vi "AddUniqueSubscription.vi"(0 "activeSubscriptions":T1[](array[typedef]), 2 "subscription":T1) -> (14 "activeSubscriptions":T1[](array[typedef]))   [LabVIEW 2017, in "STOMP.lvclass"]
uses:
  STOMP.lvclass
  Typedefs/Type_ActiveSubscription.ctl
  Typedefs/Type_AckHeader.ctl
  Typedefs/Type_FrameHeader.ctl
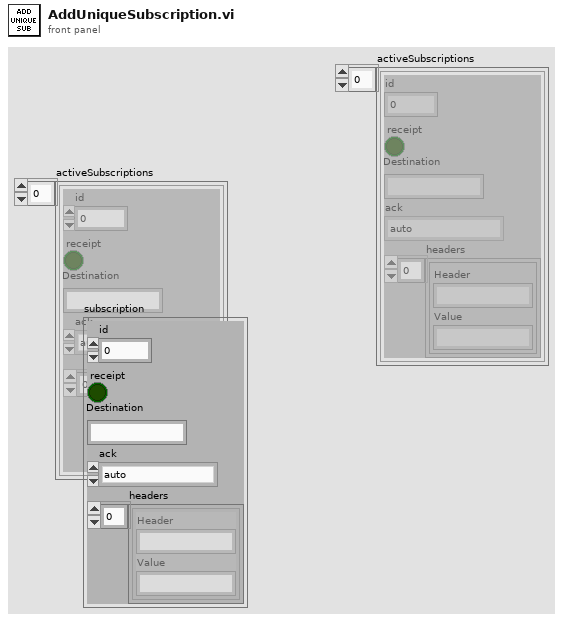
[diagram p1: front panel]
types:
  T1 = typedef "STOMP.lvclass/Type_ActiveSubscription.ctl" = cluster{"id":u64, "receipt":bool, "Destination":string, "ack":T2, "headers":T3[]}
  T2 = typedef "STOMP.lvclass/Type_AckHeader.ctl" = enum16{"auto", "client", "client-individual"}
  T3 = typedef "STOMP.lvclass/Type_FrameHeader.ctl" = cluster{"Header":string, "Value":string}
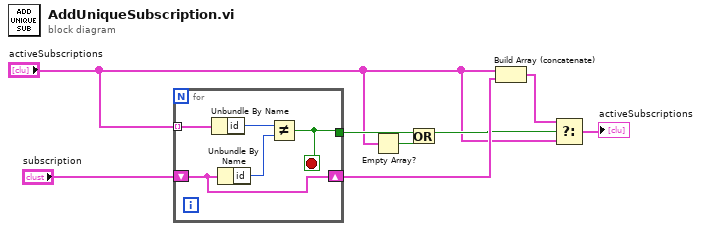
[diagram p0: block diagram]
diagram:
  n1 = for {
    tunnel: "activeSubscriptions" -> [w13] mode=indexing
    tunnel: [w10] -> w7
    shift-right: [w9] -> w6
    shift-left: "subscription" -> [w9]
    stop <- w10 stop-if-true
    n2 = Unbundle By Name(w13) -> ("id"=w12:u64)
    n3 = Unbundle By Name(w9) -> ("id"=w11:u64)
    n4 = Not Equal?(x=w12, y=w11) -> (x != y?=w10:bool)
  }
  n5 = Empty Array?(array="activeSubscriptions") -> (empty?=w2:bool)
  n6 = Or(x=w7, y=w2) -> (x .or. y?=w3:bool)
  n7 = Build Array (concatenate)("activeSubscriptions", w6) -> (w5:T1[])
  n8 = Select(t=w5, s=w3, f="activeSubscriptions") -> (s? t:f=→"activeSubscriptions":T1[])
